vi "Init OptiTrack.vi"(8 "error in (no error)":errorcluster) -> (0 "error out":errorcluster, 2 "OptiTrack Connected?":bool, 3 "Frame Grabber Data":T1)   [LabVIEW 2017]
uses:
  Controls/Tracking Data.ctl
  Controls/Packet Data.ctl
  Controls/Rigid Body Info.ctl
  Controls/Position.ctl
  Controls/Orientation.ctl
  Controls/Tracker Type.ctl
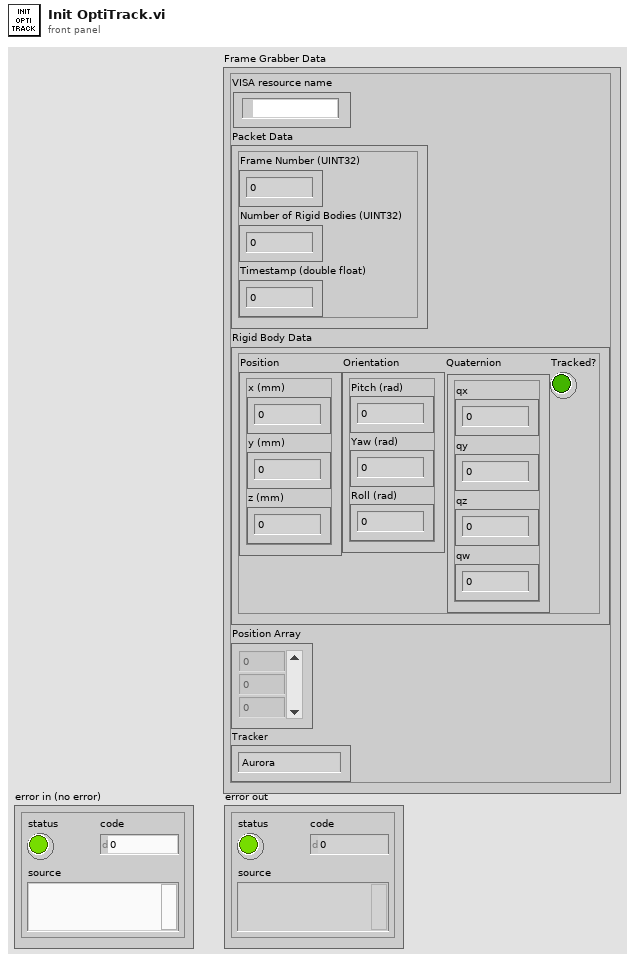
[diagram p1: front panel]
types:
  T1 = typedef "Tracking Data.ctl" = cluster{"VISA resource name":refnum<visa-resource-name>, "Packet Data":T2, "Rigid Body Data":T3, "Position Array":dbl[][], "Tracker":T6}
  T2 = typedef "Packet Data.ctl" = cluster{"Frame Number (UINT32)":u32, "Number of Rigid Bodies (UINT32)":u32, "Timestamp (double float)":dbl}
  T3 = typedef "Rigid Body Info.ctl" = cluster{"Position":T4, "Orientation":T5, "Quaternion":cluster{"qx":sgl, "qy":sgl, "qz":sgl, "qw":sgl}, "Tracked?":bool}
  T4 = typedef "Position.ctl" = cluster{"x (mm)":sgl, "y (mm)":sgl, "z (mm)":sgl}
  T5 = typedef "Orientation.ctl" = cluster{"Pitch (rad)":sgl, "Yaw (rad)":sgl, "Roll (rad)":sgl}
  T6 = typedef "Tracker Type.ctl" = enum16{"Aurora", "OptiTrack"}
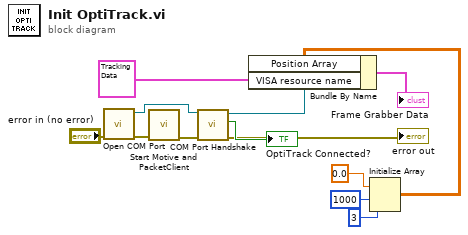
[diagram p0: block diagram]
diagram:
  n1 = call "Open COM Port.vi"("error in (no error)"="error in (no error)") -> ("error out"=w5:errorcluster, "VISA Refnum out"=w7:refnum<visa-resource-name>)  [unwired: 9 in]
  n2 = call "Start Motive and PacketClient.vi"("Error In"=w5) -> ("Error Out"=w6:errorcluster)  [unwired: 10 in]
  n3 = call "COM Port Handshake.vi"("error in (no error)"=w6, "VISA Refnum in"=w7) -> ("error out"=→"error out":errorcluster, "OptiTrack Connected?"=→"OptiTrack Connected?":bool, "VISA Refnum out"=w10:refnum<visa-resource-name>)  [unwired: 7 in]
  n4 = Initialize Array(0.0 ("element"), 1000 ("dimension size"), 3 ("dimension size")) -> (w1:dbl[][])
  n5 = Bundle By Name(cluster=T1 {"VISA resource name"="", "Packet Data"={"Frame Number (UINT32)"=0, "Number of Rigid Bodies (UINT32)"=0, "Timestamp (double float)"=0.0}, "Rigid Body Data"={"Position"={"x (mm)"=0.0, "y (mm)"=0.0, "z (mm)"=0.0}, "Orientation"={"Pitch (rad)"=0.0, "Yaw (rad)"=0.0, "Roll (rad)"=0.0}, "Quaternion"={"qx"=0.0, "qy"=0.0, "qz"=0.0, "qw"=0.0}, "Tracked?"=FALSE}, "Position Array"=[], "Tracker"=enum."Aurora"} ("Frame Grabber Data"), "Position Array"=w1, "VISA resource name"=w10) -> (→"Frame Grabber Data":T1)
